vi "MU Read Params.vi"(8 "error in (no error)":errorcluster, 11 "handle":u64) -> (0 "error out (no error)":errorcluster, 3 "function return":u32)   [LabVIEW 2017, in "MU_3SL_interface.lvlib"]
uses:
  MU_3SL_interface.lvlib
  lib/MU_3SL_interface.dll
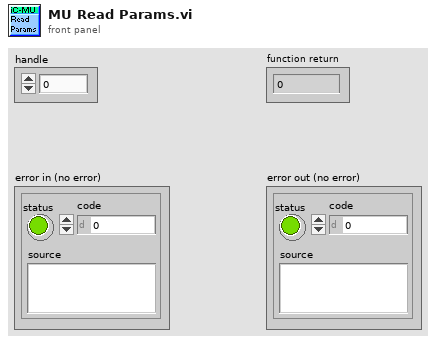
[diagram p1: front panel]
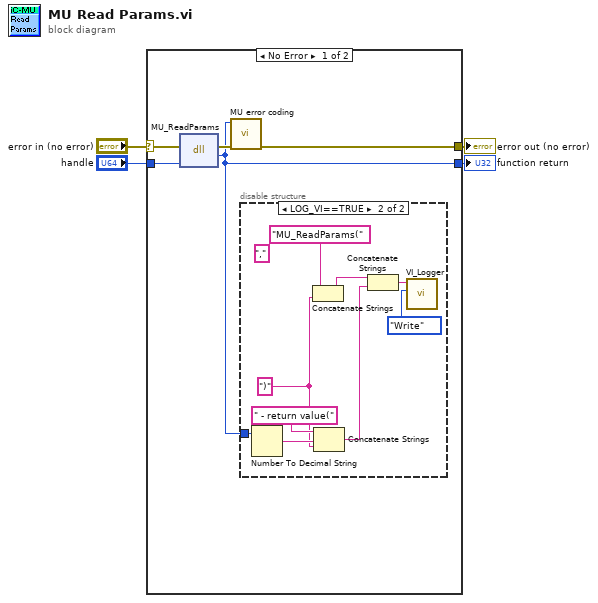
[diagram p0: block diagram]
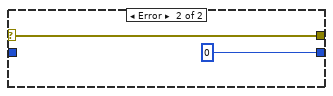
[diagram p3: hidden frame]
diagram:
  n1 = case shown="No Error" "error in (no error)" {
    selector: "error in (no error)" -> [w6 w20]
    tunnel: [w5 u32 0] -> w4
    tunnel: "handle" -> [w9 _]
    tunnel: [w7 w20] -> w2
    frame No Error {
      n2 = dll-call lib="C:/Users/bes/AppData/Roaming/work/mu_9so/icsubmodules/soft_mu_3sl_master/lv_interface/lib/MU_3SL_interface**.*" fn="MU_ReadParams"(error in=w6, "handle"=w9) -> (error out=w8:errorcluster, "return type"=w5:u32)  [unwired: 3 in, 1 out]
      n3 = call "MU error coding.vi"("error in (no error)"=w8, "function return in"=w5) -> ("error out"=w7:errorcluster)  [unwired: 9 in]
      n4 = disable-structure shown="LOG_VI==TRUE" {
        disable-tunnel: w5 -> [_ w16]
        frame condition #0 {
        }
        frame condition #1 (active) {
          w10 = ")" ("string")
          (unwired) "," ("string")
          n5 = Number To Decimal String(number=w16) -> (decimal integer string=w15:string)  [unwired: 1 in]
          n6 = Concatenate Strings("MU_ReadParams(" ("Info in"), w10) -> (w14:string)
          n7 = Concatenate Strings(" - return value(" ("string"), w15, w10) -> (w13:string)
          n8 = Concatenate Strings(w14, w13) -> (w12:string)
          n9 = call "VI_Logger.vi"("Action (Read)"=enum16{"Write", "Read"}."Write", "Info in"=w12) -> ()  [unwired: 8 in, 2 out]
        }
      }
    }
    frame Error {
    }
  }
  "function return" <- w4
  "error out (no error)" <- w2
